vi "Main.vi"(11 "_Template in":refnum<class "_Template.lvclass">) -> (0 "error out":errorcluster, 3 "_Template out":refnum<class "_Template.lvclass">)   [LabVIEW 2020, in "_Template.lvlib" / "_Template.lvclass"]
uses:
  _Template.lvclass
  _Template.lvclass/_Template.ctl
  _Shared/Project Stuff/Project Stuff.lvclass
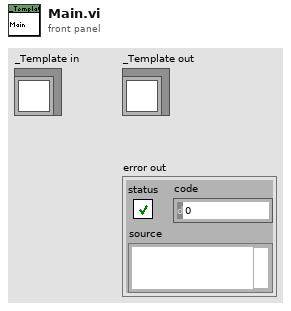
[diagram p1: front panel]
types:
  T1 = typedef "_Shared.lvlib/Project Stuff.lvclass/Refs.ctl" = cluster{"Target":refnum<vi>, "VI":T2, "Library":T3}
  T2 = typedef "_Shared.lvlib/Project Stuff.lvclass/VI.ctl" = set{refnum<vi>}
  T3 = typedef "_Shared.lvlib/Project Stuff.lvclass/Library.ctl" = set{refnum<vi>}
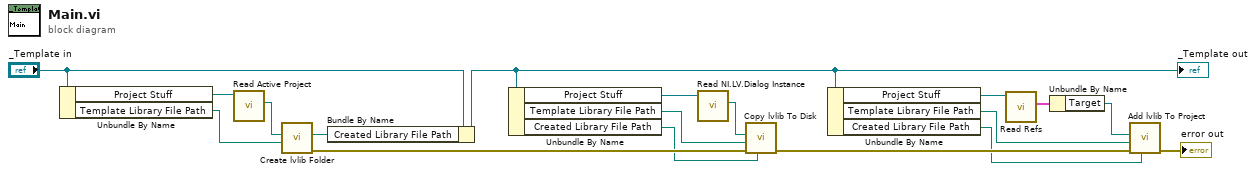
[diagram p0: block diagram]
diagram:
  n1 = Unbundle By Name("_Template in") -> ("Project Stuff"=w8:refnum<class "Project Stuff.lvclass">, "Template Library File Path"=w14:path)
  n2 = call "Read Active Project.vi"("Project Stuff in"=w8) -> ("Active Project"=w7:refnum<vi>)  [unwired: 10 in]
  n3 = call "Create lvlib Folder.vi"("Template Library File Path"=w14, "Active Project"=w7) -> ("error out"=w13:errorcluster, "Created Library File Path"=w15:path)  [unwired: 8 in]
  n4 = Bundle By Name(cluster="_Template in", "Created Library File Path"=w15) -> (w4:refnum<class "_Template.lvclass">)
  "_Template out" <- w4
  n5 = Unbundle By Name(w4) -> ("Project Stuff"=w6:refnum<class "Project Stuff.lvclass">, "Template Library File Path"=w18:path, "Created Library File Path"=w12:path)
  n6 = call "Read NI.LV.Dialog Instance.vi"("Project Stuff in"=w6) -> ("NI.LV.Dialog Instance"=w5:refnum<vi>)  [unwired: 10 in]
  n7 = call "Copy lvlib To Disk.vi"("Created Library File Path"=w12, "error in"=w13, "Template Library File Path"=w18, "NI.LV.Dialog Instance"=w5) -> ("error out"=w17:errorcluster)  [unwired: 7 in]
  n8 = Unbundle By Name(w4) -> ("Project Stuff"=w3:refnum<class "Project Stuff.lvclass">, "Template Library File Path"=w10:path, "Created Library File Path"=w11:path)
  n9 = call "Read Refs.vi"("Project Stuff in"=w3) -> ("Refs"=w2:T1)  [unwired: 10 in]
  n10 = Unbundle By Name(w2) -> ("Target"=w1:refnum<vi>)
  n11 = call "Add lvlib To Project.vi"("Created Library File Path"=w11, "error in"=w17, "Template Library File Path"=w10, "Target"=w1) -> ("error out"=→"error out":errorcluster)  [unwired: 7 in]
